vi "Resolve VI Refnum.vi"(8 "error in (no error)":errorcluster, 10 "VI Name":string, 11 "VI Refnum":refnum<vi>) -> (0 "error out":errorcluster, 3 "UI Refnum":refnum<vi>)   [LabVIEW 2014]
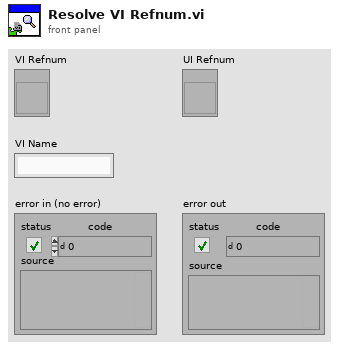
[diagram p1: front panel]
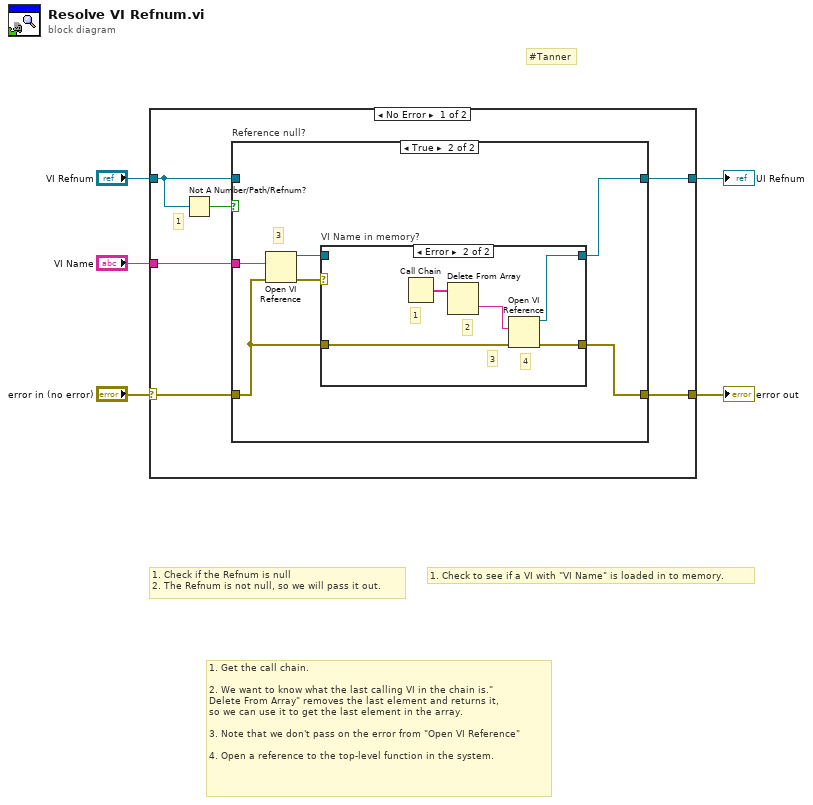
[diagram p0: block diagram]
diagram:
  # "#Tanner"
  # "1. Get the call chain.\n\n2. We want to know what the last calling VI in the chain is.\" \nDelete From Array\" removes the last element and returns it, \nso we can use it to get the last element in the array.\n\n3. Note that we don't pass on the error from \"Open VI Reference\"\n\n4. Open a reference to the top-level function in the system."
  # "1. Check to see if a VI with \"VI Name\" is loaded in to memory."
  # "1. Check if the Refnum is null\n2. The Refnum is not null, so we will pass it out."
  n1 = case shown="No Error" "error in (no error)" {
    selector: "error in (no error)" -> [w7 w27]
    tunnel: "VI Name" -> [w8 _]
    tunnel: "VI Refnum" -> [w10 w28]
    tunnel: [w9 w28] -> w2
    tunnel: [w6 w27] -> w1
    frame No Error {
      # "1"
      n2 = Not A Number/Path/Refnum?(number/path/refnum=w10) -> (NaN/Path/Refnum?=w11:bool)
      n3 = case "Reference null?" shown="True" w11 {
        tunnel: w10 -> [w13 _]
        tunnel: [w13 w17] -> w9
        tunnel: w8 -> [_ w19]
        tunnel: w7 -> [w12 w15]
        tunnel: [w12 w14] -> w6
        frame False {
          # "2"
        }
        frame True {
          # "3"
          n4 = Open VI Reference(vi path=w19, error in (no error)=w15) -> (vi reference=w16:refnum<vi>, error out=w18:errorcluster)  [unwired: 4 in]
          n5 = case "VI Name in memory?" shown="Error" w18 {
            tunnel: [w21 w24] -> w17
            tunnel: w16 -> [w21 _]
            tunnel: w15 -> [w20 w23]
            tunnel: [w20 w22] -> w14
            frame No Error {
            }
            frame Error {
              # "4"
              # "3"
              # "2"
              # "1"
              n6 = Call Chain() -> (call chain=w26:string[])
              n7 = Delete From Array(array=w26) -> (deleted portion=w25:string)  [unwired: 2 in, 1 out]
              n8 = Open VI Reference(vi path=w25, error in (no error)=w23) -> (vi reference=w24:refnum<vi>, error out=w22:errorcluster)  [unwired: 4 in]
            }
          }
        }
      }
    }
    frame Error {
    }
  }
  "error out" <- w1
  "UI Refnum" <- w2
